vi "ViewImageSetnew.vi"(1 "Cluster":T4 {"?" format="%.2f"; "?"."?" format="%.2f"; "?"."?" format="%.2f"; "?"."?" format="%.2f"; "?"."?" format="%.2f"; "?"."?" format="%.2f"; "?"."?" format="%.2f"; "?"."?" format="%.2f"; "?"."?" format="%.2f"; "?"."?" format="%.2f"; "?"."?" format="%.2f"; "?"."?" format="%.2f"; "?"."?" format="%.2f"}, 2 "Path":path, 3 "action":T5(ring)) -> (0 "Image Settings":T1={"Start Position (µm)"={"x"=0.0, "y"=0.0, "z"=0.0}, "End Position (µm)"={"x"=10.0, "y"=10.0, "z"=0.0}, "Image Resolution (nm/pixel)"={"x"=50.0, "y"=50.0, "z"=100.0}, "Image Size (µm)"={"x"=10.0, "y"=10.0, "z"=0.0}, "Image Size (pixel)"={"x"=50, "y"=50, "z"=0}, "Time Resolution\n(ms/pixel)"=7.0, "1st Axis"=0, "2nd Axis"=1, "Retrace"=FALSE, "Estimated Time"=""} {"2nd Axis" items=["x", "y", "z"]; "1st Axis" items=["x", "y", "z"]; "Time Resolution\n(ms/pixel)" format="%.2f"; "Image Resolution (nm/pixel)"."z" format="%.2f"; "Image Resolution (nm/pixel)"."y" format="%.2f"; "Image Resolution (nm/pixel)"."x" format="%.2f"; "Image Size (µm)"."z" format="%.2f"; "Image Size (µm)"."y" format="%.2f"; "Image Size (µm)"."x" format="%.2f"; "End Position (µm)"."z" format="%.2f"; "End Position (µm)"."y" format="%.2f"; "End Position (µm)"."x" format="%.2f"; "Start Position (µm)"."z" format="%.2f"; "Start Position (µm)"."y" format="%.2f"; "Start Position (µm)"."x" format="%.2f"})   [LabVIEW 2009]
uses:
  ImageSettings.ctt
  FIFOSettings_BH.ctt
  <vilib>/Utility/xml.llb/Read From XML File(string).vi
panel:
  in  "output cluster":T3 {"Image Settings"."2nd Axis" items=["x", "y", "z"]; "Image Settings"."1st Axis" items=["x", "y", "z"]; "Image Settings"."Time Resolution\n(ms/pixel)" format="%.2f"; "Image Settings"."Image Resolution (nm/pixel)"."z" format="%.2f"; "Image Settings"."Image Resolution (nm/pixel)"."y" format="%.2f"; "Image Settings"."Image Resolution (nm/pixel)"."x" format="%.2f"; "Image Settings"."Image Size (µm)"."z" format="%.2f"; "Image Settings"."Image Size (µm)"."y" format="%.2f"; "Image Settings"."Image Size (µm)"."x" format="%.2f"; "Image Settings"."End Position (µm)"."z" format="%.2f"; "Image Settings"."End Position (µm)"."y" format="%.2f"; "Image Settings"."End Position (µm)"."x" format="%.2f"; "Image Settings"."Start Position (µm)"."z" format="%.2f"; "Image Settings"."Start Position (µm)"."y" format="%.2f"; "Image Settings"."Start Position (µm)"."x" format="%.2f"; "FIFO Settings"."CFD"."CFD Holdoff (ns)" min=5 max=20 format="%.2f"; "FIFO Settings"."CFD"."CFD ZC Level (mV)" min=-96 max=96 format="%.2f"; "FIFO Settings"."CFD"."CFD Limit High (mV)" min=4 max=80 format="%.2f"; "FIFO Settings"."CFD"."CFD Limit Low (mV)" min=-500 max=80 format="%.2f"; "FIFO Settings"."TAC"."TAC Limit High (%)" min=0 max=100 format="%.2f"; "FIFO Settings"."TAC"."TAC Limit Low (%)" min=0 max=100 format="%.2f"; "FIFO Settings"."TAC"."TAC Offset (%)" min=0 max=100 format="%.2f"; "FIFO Settings"."TAC"."TAC Gain" min=1 max=15 step=1; "FIFO Settings"."TAC"."TAC Range (ns)" min=50 max=2000 format="%.2f"; "FIFO Settings"."SYNC"."SYNC Threshold (mV)" min=-500 max=-19 format="%.2f"; "FIFO Settings"."SYNC"."SYNC Holdoff (ns)" min=4 max=16 format="%.2f"; "FIFO Settings"."SYNC"."SYNC Freq Divider" min=1 max=16 step=1; "FIFO Settings"."SYNC"."SYNC ZC Level (mV)" min=-96 max=96 format="%.2f"; "FIFO Settings"."ADC"."Macro Time Clock" items=["Internal (50ns)", "Sync-Trigger", "1/2 Sync-Trigger"]; "FIFO Settings"."ADC"."Module" items=["SPC 630", "SPC 830", "SPC 13x", "HydraHarp"]; "FIFO Settings"."ADC"."Count Increment" min=1 max=255 step=1; "FIFO Settings"."ADC"."Dither Range" min=0 max=256 step=32; "FIFO Settings"."Measurement"."Ext Latch Delay" min=0 max=255 step=1; "FIFO Settings"."Measurement"."Stop Count" format="%.2f"; "FIFO Settings"."Measurement"."Stop Condition:" items=["None", "Photon Count", "Time (s)"]; "FIFO Settings"."Measurement"."External Trigger Condition" max=2 step=1; "FIFO Settings"."Measurement"."No of Channels" max=14; "FIFO Settings"."Measurement"."Binning (ms)" min=1e-07 max=100000 format="%.3f"}
  in  "OK Button":bool
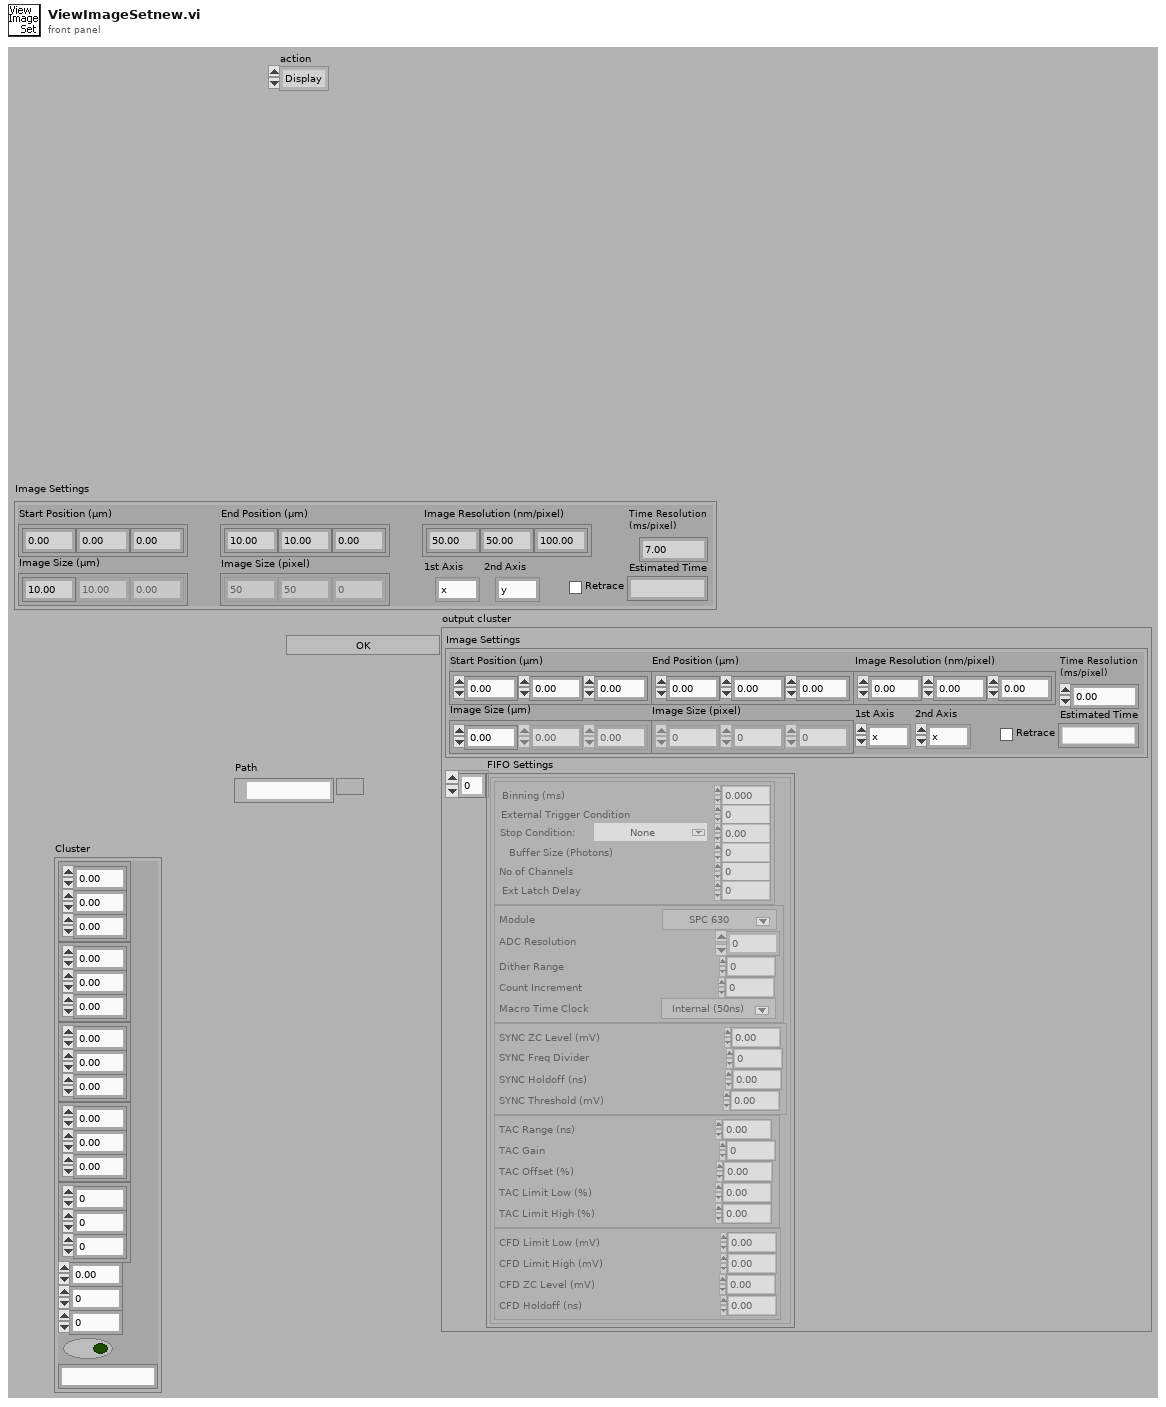
[diagram p1: front panel]
types:
  T1 = typedef "ImageSettings.ctt" = cluster{"Start Position (µm)":cluster{"x":dbl, "y":dbl, "z":dbl}, "End Position (µm)":cluster{"x":dbl, "y":dbl, "z":dbl}, "Image Resolution (nm/pixel)":cluster{"x":dbl, "y":dbl, "z":dbl}, "Image Size (µm)":cluster{"x":dbl, "y":dbl, "z":dbl}, "Image Size (pixel)":cluster{"x":u32, "y":u32, "z":u32}, "Time Resolution\n(ms/pixel)":dbl, "1st Axis":u16, "2nd Axis":u16, "Retrace":bool, "Estimated Time":string}
  T2 = typedef "FIFOSettings_BH.ctt" = cluster{"Measurement":cluster{"Binning (ms)":sgl, "External Trigger Condition":u16, "Stop Condition:":u16, "Stop Count":dbl, "Buffer Size (Photons)":u16, "No of Channels":u16, "Ext Latch Delay":i16}, "ADC":cluster{"Module":u16, "ADC Resolution":i32, "Dither Range":i16, "Count Increment":i16, "Macro Time Clock":i16}, "SYNC":cluster{"SYNC ZC Level (mV)":sgl, "SYNC Freq Divider":i16, "SYNC Holdoff (ns)":sgl, "SYNC Threshold (mV)":sgl}, "TAC":cluster{"TAC Range (ns)":sgl, "TAC Gain":i16, "TAC Offset (%)":sgl, "TAC Limit Low (%)":sgl, "TAC Limit High (%)":sgl}, "CFD":cluster{"CFD Limit Low (mV)":sgl, "CFD Limit High (mV)":sgl, "CFD ZC Level (mV)":sgl, "CFD Holdoff (ns)":sgl}}
  T3 = cluster{"Image Settings":T1, "FIFO Settings":T2[]}
  T4 = cluster{cluster{dbl, dbl, dbl}, cluster{dbl, dbl, dbl}, cluster{dbl, dbl, dbl}, cluster{dbl, dbl, dbl}, cluster{u32, u32, u32}, dbl, u16, u16, bool, string}
  T5 = enum16{"Display", "change", "Get", "Set", "Set Ken"}
  T6 = cluster{"Image Settings":T1, cluster{"Measurement":cluster{"Binning (ms)":sgl, "External Trigger Condition":u16, "Stop Condition:":u16, "Stop Count":dbl, "Buffer Size (Photons)":u16, "No of Channels":u16, "Ext Latch Delay":i16}, "ADC":cluster{"Module":u16, "ADC Resolution":i32, "Dither Range":i16, "Count Increment":i16, "Macro Time Clock":i16}, "SYNC":cluster{"SYNC ZC Level (mV)":sgl, "SYNC Freq Divider":i16, "SYNC Holdoff (ns)":sgl, "SYNC Threshold (mV)":sgl}, "TAC":cluster{"TAC Range (ns)":sgl, "TAC Gain":i16, "TAC Offset (%)":sgl, "TAC Limit Low (%)":sgl, "TAC Limit High (%)":sgl}, "CFD":cluster{"CFD Limit Low (mV)":sgl, "CFD Limit High (mV)":sgl, "CFD ZC Level (mV)":sgl, "CFD Holdoff (ns)":sgl}}[]}
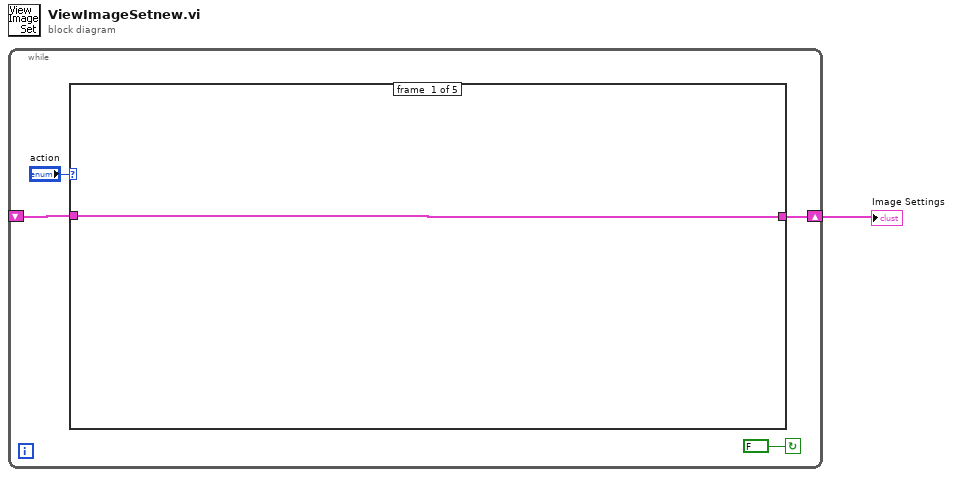
[diagram p0: block diagram]
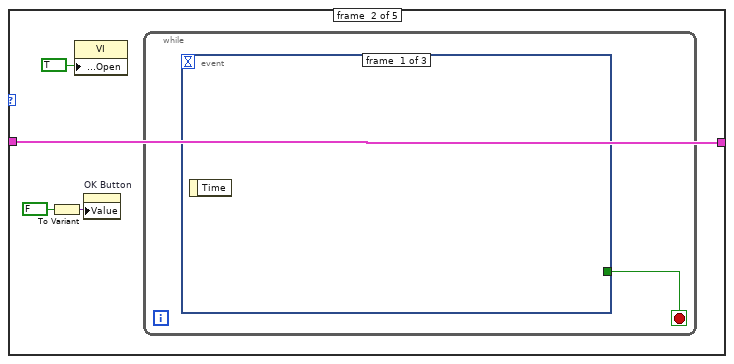
[diagram p2: hidden frame]
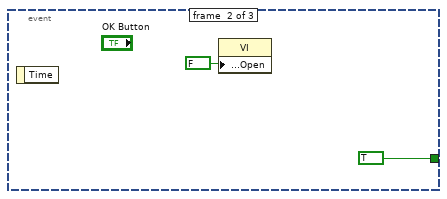
[diagram p3: hidden frame]
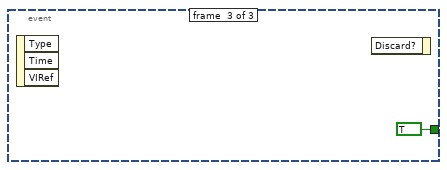
[diagram p4: hidden frame]
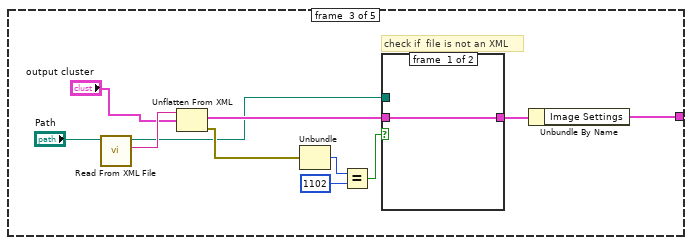
[diagram p5: hidden frame]
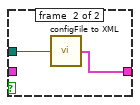
[diagram p6: hidden frame]
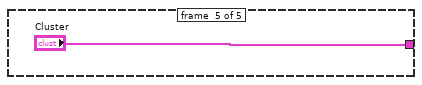
[diagram p8: hidden frame]
diagram:
  n1 = while {
    shift-right: [w3] -> w1
    shift-left: _ -> [w4]
    stop <- FALSE continue-if-true
    n2 = case shown="\"Set\"" "action" {
      tunnel: w4 -> [w6 w9 _ w28 _]
      tunnel: [w6 w9 w15 w28 "Cluster"] -> w3
      frame #0 {
      }
      frame #1 {
        n3 = To Variant(anything=FALSE) -> (Variant=w7:variant)
        n4 = property class="VI"("Front Panel Window:Open"=TRUE) -> ()  [unwired: 2 in, 2 out]
        n5 = property on="OK Button" class="Bool"("Value"=w7) -> ()  [unwired: 2 in, 2 out]
        n6 = while {
          stop <- w11 stop-if-true
          n7 = event shown="[2] Panel Close?" {
            selector: _ -> [_ _ _]
            dyn-events: _ -> [_ _ _]
            timeout: _ -> [_ _ _]
            tunnel: [_ TRUE TRUE] -> w11
            event #0 {
              n8 = event-data() -> ()  [unwired: 1 in, 1 out]
            }
            event #1 {
              n9 = event-data() -> ()  [unwired: 1 in, 1 out]
              n10 = property class="VI"("Front Panel Window:Open"=FALSE) -> ()  [unwired: 2 in, 2 out]
            }
            event #2 {
              n11 = event-data() -> ()  [unwired: 1 in, 3 out]
              n12 = event-data() -> ()  [unwired: 2 in, 1 out]
            }
          }
        }
      }
      frame #2 {
        # "check if  file is not an XML"
        n13 = call-poly <vilib>:"Read From XML File.vi"("XML File Path"="Path") -> ("XML Elements"=w24:string)  [unwired: 8 in, 2 out]
        n14 = Unflatten From XML(xml string=w24, type="output cluster") -> (value=w17:T3, error out=w18:errorcluster)  [unwired: 1 in]
        n15 = Unbundle(w18) -> ("code"=w22:i32)  [unwired: 2 out]
        n16 = Equal?(x=w22, y=1102) -> (x = y?=w20:bool)
        n17 = case shown="False" w20 {
          tunnel: [w25 w26] -> w19
          tunnel: w17 -> [w25 _]
          tunnel: "Path" -> [_ w27]
          frame #0 {
          }
          frame #1 {
            n18 = call "configFile to XML.vi"("configuration file path"=w27) -> ("output cluster"=w26:T6)
          }
        }
        n19 = Unbundle By Name(w19) -> ("Image Settings"=w15:T1)
      }
      frame #3 {
      }
      frame #4 {
      }
    }
  }
  "Image Settings" <- w1
